vi "Arrays.vi"() -> ()   [LabVIEW 2021]
panel:
  in  "index":i32
  out "element":dbl
  out "size(s)":i32
  in  "Array 4":bool[](array[boolean])
  out "Array 3":bool[](array[boolean])
  out "Array 2":dbl[](array[slide]) scale=0.0..10.0
  in  "Array":dbl[](array[numeric])
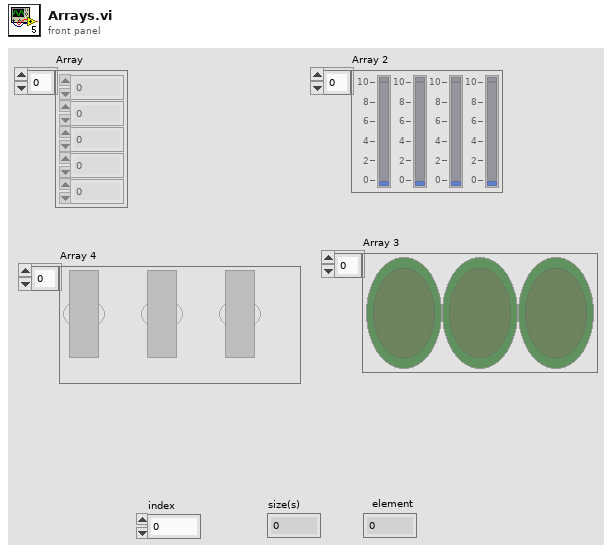
[diagram p1: front panel]
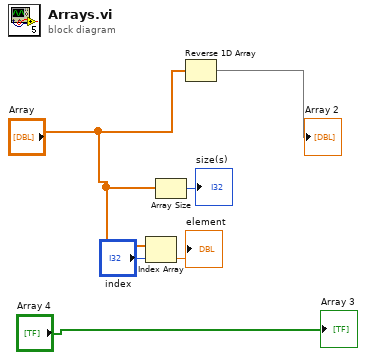
[diagram p0: block diagram]
diagram:
  n1 = Index Array(array="Array", index="index") -> (element=→"element":dbl)
  n2 = Array Size(array="Array") -> (size(s)=→"size(s)":i32)
  n3 = Reverse 1D Array(array="Array") -> (reversed array=→"Array 2":dbl[])
  "Array 3" <- "Array 4"
